vi "sensory_mapping.vi"() -> ()   [LabVIEW 2017]
uses:
  <resource>/objmgr/daqmx.rc
  <vilib>/DAQmx/create/channels.llb/DAQmx Create Channel (DO-Digital Output).vi
  <vilib>/DAQmx/write.llb/DAQmx Write (Digital Bool 1Line 1Point).vi
  const.ctl
  <vilib>/Waveform/WDTOps.llb/WDT Get Waveform Time Array DBL.vi
  <vilib>/DAQmx/read.llb/DAQmx Read (Analog Wfm 1Chan 1Samp).vi
  <vilib>/DAQmx/configure/timing.llb/DAQmx Timing (Sample Clock).vi
  <vilib>/DAQmx/create/channels.llb/DAQmx Create Channel (AI-Voltage-Basic).vi
  <vilib>/Utility/file.llb/Write Delimited Spreadsheet (DBL).vi
  <vilib>/Utility/file.llb/Write Delimited Spreadsheet (string).vi
panel:
  in  "Session":i32=1
  in  "Mouse ID":string
  in  "Base data directory":path
  in  "Stimulated brain region":string
  in  "Vibration Amplitude":dbl
  in  "Vibration frequency (Hz)":dbl
  in  "Simulus duration (seconds)":dbl
  in  "Repeats":i16
  in  "Post_stim (s)":dbl
  in  "Pre_stim (s)":dbl
  in  "Investigator":string
  in  "Stim Type":enum16{"Visual", "Sensory", "Auditory"}(ring)=enum."Sensory"
  in  "Tone Frequency (Hz)":dbl
  out "Stim times":dbl[](array[numeric])
  in  "stop":bool
  out "Current stim iteration":i32
  out "Measured Stim duration (s)":dbl
  in  "Sensory stim output line":tag="Dev3/port1/line3"
  in  "Analog input lines":tag="Dev3/ai0"
  in  "LED output line":tag="Dev3/port1/line1"
  out "Stop time (seconds)":dbl
  out "Stim status":bool
  out "Time from sample clock":dbl
  out "Camera exposure signals":waveform(dbl)(graph)
  out "Sampling rate (Hz)":dbl
  # "Timing parameters"
  # "Stim parameters"
  # "n.b. the params below are changed by the stim box\nthey are not controlled by this VI"
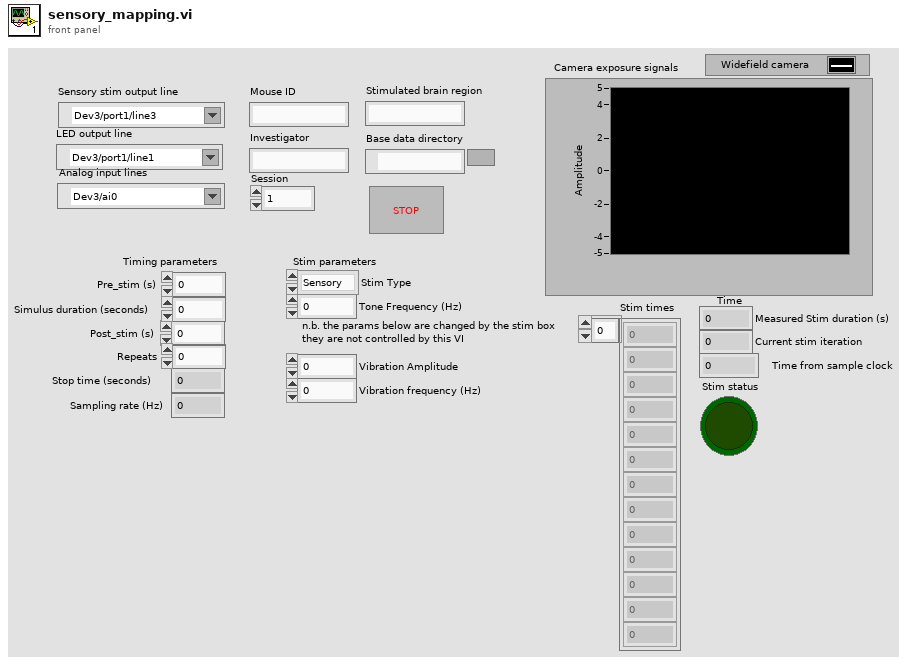
[diagram p1: front panel]
types:
  T1 = cluster{"Mouse ID":string, "Visual Timestamps":dbl[], "Sensory Timestamps":dbl[], "Investigator":string, "Auditory Timestamps":dbl[], "Stim Type":string, "Stop Time":dbl, "Sampling Rate":dbl, "Stimulus Duration (s)":dbl, "Tone Frequency":dbl, "Date_Time":string, "Session":i16, "Synchronisation":dbl[][], "Stimulated brain region":string, "Repeats":i32, "Pre_stim (s)":dbl, "Post_stim (s)":dbl, "Vibration Amplitude":dbl, "Vibration frequency(Hz)":dbl}
  T2 = typedef "const.ctl" = cluster{"Visual":refnum<queue>, "Sensory":refnum<queue>, "Auditory":refnum<queue>}
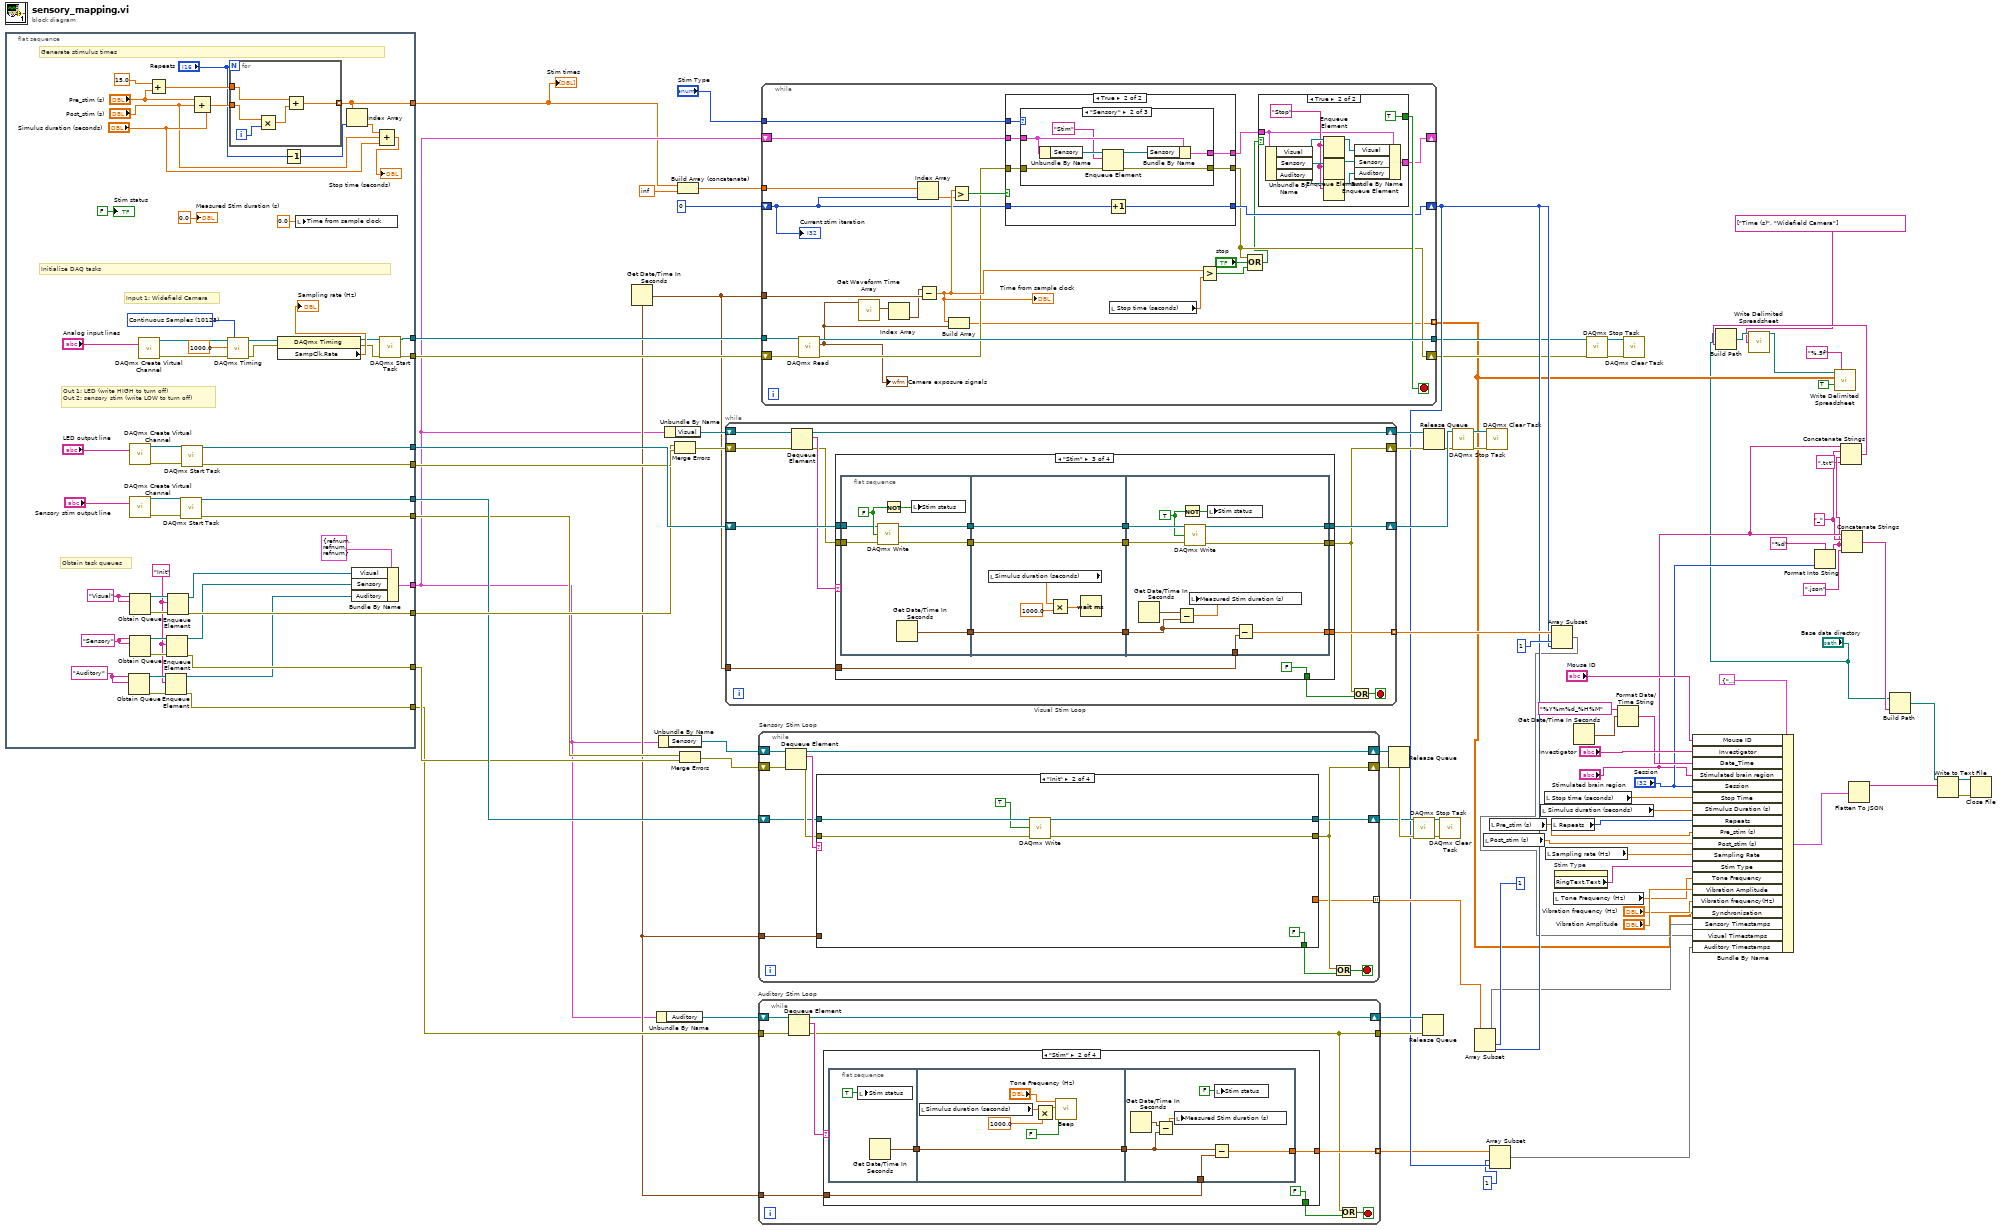
[diagram p0: block diagram]
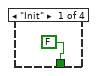
[diagram p2: hidden frame]
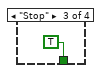
[diagram p3: hidden frame]
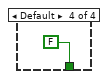
[diagram p4: hidden frame]
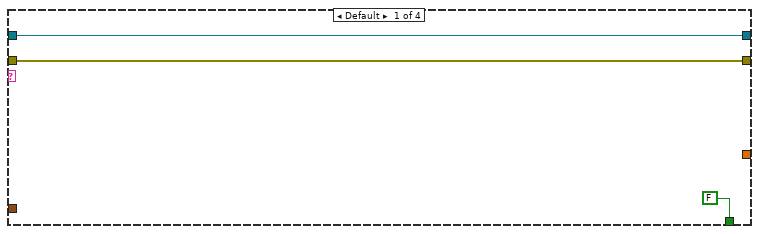
[diagram p5: hidden frame]
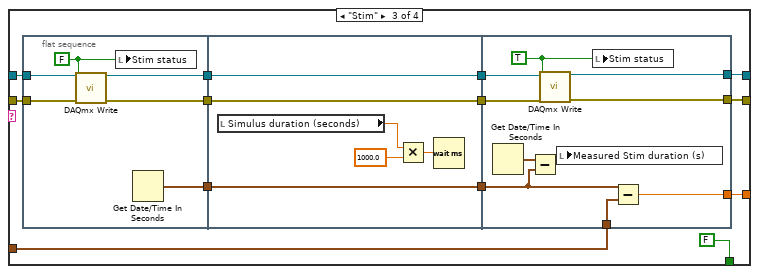
[diagram p6: hidden frame]
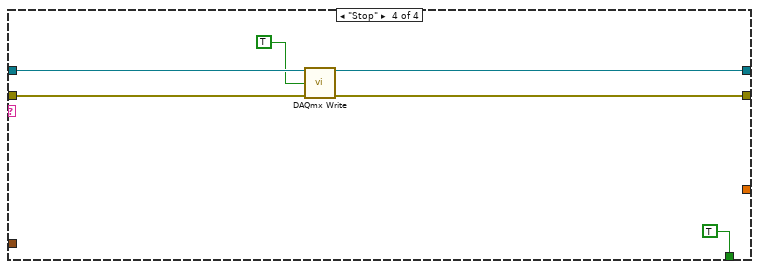
[diagram p7: hidden frame]
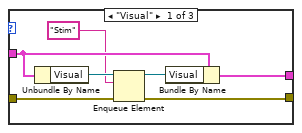
[diagram p9: hidden frame]
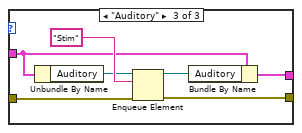
[diagram p10: hidden frame]
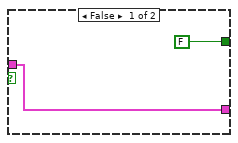
[diagram p11: hidden frame]
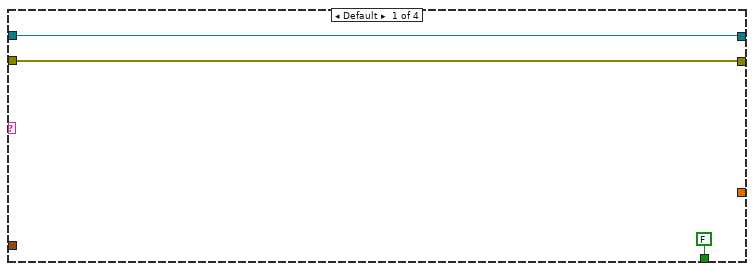
[diagram p12: hidden frame]
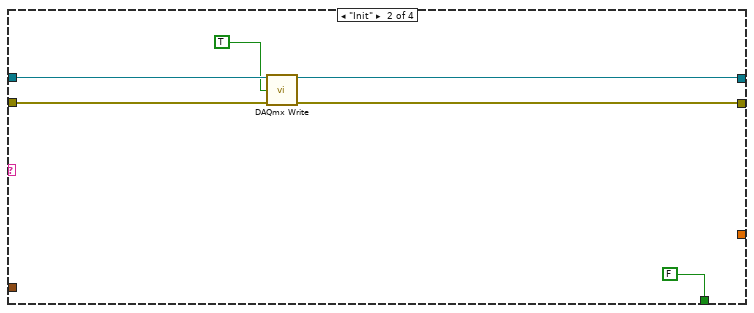
[diagram p13: hidden frame]
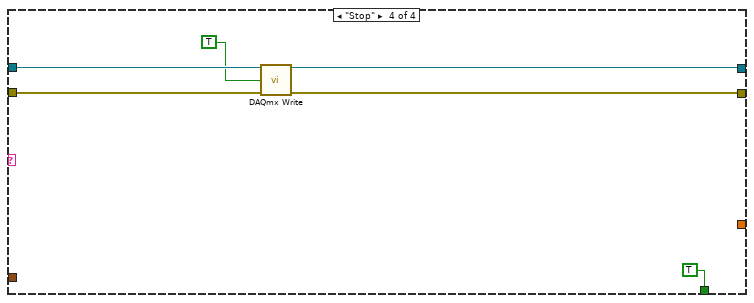
[diagram p14: hidden frame]
diagram:
  w7 = "_" ("string")
  n1 = flat-sequence {
    tunnel: [w127] -> w76
    tunnel: [w126] -> w75
    tunnel: [w122] -> w86
    tunnel: [w121] -> w80
    tunnel: [w117] -> w69
    tunnel: [w109] -> w63
    tunnel: [w108] -> w57
    tunnel: [w103] -> w52
    tunnel: [w102] -> w65
    tunnel: [w101] -> w64
    tunnel: [w93] -> w37
    frame #0 {
      w115 = "Auditory" ("name (unnamed)")
      w116 = "Sensory" ("name (unnamed)")
      w110 = "Init" ("element")
      w118 = "Visual" ("name (unnamed)")
      w138 = 10123 items=["Finite Samples"=10178, "Continuous Samples"=10123, "Hardware Timed Single Point"=12522] ("sample mode")
      # "Generate stimulus times"
      # "Obtain task queues"
      # "Initialize DAQ tasks"
      # "Input 1: Widefield Camera"
      # "Out 1: LED (write HIGH to turn off)\nOut 2: sensory stim (write LOW to turn off)"
      n2 = Obtain Queue(name (unnamed)=w115, element data type=w115) -> (queue out=w112:refnum<queue>, error out=w111:errorcluster)  [unwired: 3 in, 1 out]
      n3 = call-poly <vilib>:"DAQmx Create Virtual Channel.vi"("lines"="LED output line") -> ("task out"=w137:refnum<k21>, "error out"=w136:errorcluster)  [unwired: 13 in]
      n4 = call-poly <vilib>:"DAQmx Create Virtual Channel.vi"("lines"="Sensory stim output line") -> ("task out"=w124:refnum<k21>, "error out"=w123:errorcluster)  [unwired: 13 in]
      n5 = Obtain Queue(name (unnamed)=w118, element data type=w118) -> (queue out=w119:refnum<queue>, error out=w120:errorcluster)  [unwired: 3 in, 1 out]
      n6 = Obtain Queue(name (unnamed)=w116, element data type=w116) -> (queue out=w114:refnum<queue>, error out=w113:errorcluster)  [unwired: 3 in, 1 out]
      n7 = call-poly <vilib>:"DAQmx Create Virtual Channel.vi"("physical channels"="Analog input lines") -> ("task out"=w139:refnum<k21>, "error out"=w140:errorcluster)  [unwired: 13 in]
      n8 = Add(x=15.0, y="Pre_stim (s)") -> (x+y=w94:dbl)
      n9 = Enqueue Element(queue=w112, element=w110, error in (no error)=w111) -> (queue out=w104:refnum<queue>, error out=w108:errorcluster)  [unwired: 1 in, 1 out]
      n10 = Enqueue Element(queue=w114, element=w110, error in (no error)=w113) -> (queue out=w105:refnum<queue>, error out=w109:errorcluster)  [unwired: 1 in, 1 out]
      n11 = Enqueue Element(queue=w119, element=w110, error in (no error)=w120) -> (queue out=w106:refnum<queue>, error out=w117:errorcluster)  [unwired: 1 in, 1 out]
      n12 = call <vilib>:"DAQmx Start Task.vi"("task/channels in"=w124, "error in"=w123) -> ("task out"=w102:refnum<k21>, "error out"=w101:errorcluster)  [unwired: 12 in]
      n13 = call <vilib>:"DAQmx Start Task.vi"("task/channels in"=w137, "error in"=w136) -> ("task out"=w122:refnum<k21>, "error out"=w121:errorcluster)  [unwired: 12 in]
      n14 = Compound Arithmetic op=ADD("Pre_stim (s)", "Post_stim (s)", "Simulus duration (seconds)") -> (w97:dbl)
      n15 = call-poly <vilib>:"DAQmx Timing.vi"("task/channels in"=w139, "sample mode"=w138, "rate"=1000.0, "error in"=w140) -> ("task out"=w132:refnum<k21>, "error out"=w131:errorcluster)  [unwired: 10 in]
      n16 = for {
        N: "Repeats" -> [_]
        tunnel: w97 -> [w144]
        tunnel: w94 -> [w143]
        tunnel: [w141] -> w93 mode=indexing
        i -> [w145]
        n17 = Multiply(x=w144, y=w145) -> (x*y=w142:dbl)
        n18 = Add(x=w143, y=w142) -> (x+y=w141:dbl)
      }
      n19 = property class="DAQmx Timing"(reference=w132, error in=w131) -> (reference out=w129:refnum<k21>, error out=w128:errorcluster, "SampClk.Rate"=→"Sampling rate (Hz)":dbl)
      n20 = Decrement(x="Repeats") -> (x-1=w91:i16)
      n21 = local write "Time from sample clock"(0.0 ("Time from sample clock")) -> ()
      n22 = Index Array(array=w93, index=w91) -> (element=w90:dbl)
      n23 = Bundle By Name(cluster=T2 {"Visual"=refnum, "Sensory"=refnum, "Auditory"=refnum}, "Visual"=w106, "Sensory"=w105, "Auditory"=w104) -> (w103:T2)
      n24 = Compound Arithmetic op=ADD(w90, "Post_stim (s)", "Simulus duration (seconds)") -> (→"Stop time (seconds)":dbl)
      n25 = call <vilib>:"DAQmx Start Task.vi"("task/channels in"=w129, "error in"=w128) -> ("task out"=w127:refnum<k21>, "error out"=w126:errorcluster)  [unwired: 12 in]
      "Stim status" <- FALSE ("LED status")
      "Measured Stim duration (s)" <- 0.0 ("Measured LED duration")
    }
  }
  n26 = Get Date/Time In Seconds() -> (seconds since 1Jan1904=w54:timestamp)
  n27 = Unbundle By Name(w52) -> ("Auditory"=w56:refnum<queue>)
  n28 = Unbundle By Name(w52) -> ("Sensory"=w66:refnum<queue>)
  n29 = Unbundle By Name(w52) -> ("Visual"=w68:refnum<queue>)
  n30 = Merge Errors(w69, w80) -> (w79:errorcluster)
  n31 = Build Array (concatenate)(w37, inf) -> (w74:dbl[])
  n32 = Merge Errors(w64, w63) -> (w62:errorcluster)
  n33 = while "Visual Stim Loop" {
    tunnel: [w157] -> w70 mode=indexing
    shift-right: [w155] -> w81
    shift-left: w86 -> [w156]
    shift-right: [w152] -> w78
    shift-left: w79 -> [w151]
    shift-right: [w146] -> w67
    shift-left: w68 -> [w147]
    tunnel: w54 -> [w148]
    stop <- w154 stop-if-true
    n34 = Dequeue Element(queue=w147, error in (no error)=w151) -> (queue out=w146:refnum<queue>, element=w150:string, error out=w149:errorcluster)  [unwired: 1 in, 1 out]
    n35 = case shown="\"Stim\"" w150 {
      tunnel: [_ _ w173 _] -> w157
      tunnel: w156 -> [w160 w166 w172 w209]
      tunnel: w149 -> [w159 w165 w171 w208]
      tunnel: [w160 w164 w170 w206] -> w155
      tunnel: [w159 w163 w169 w205] -> w152
      tunnel: [FALSE FALSE FALSE TRUE] -> w153
      tunnel: w148 -> [_ _ w167 _]
      frame Default {
      }
      frame "Init" {
        n36 = call-poly <vilib>:"DAQmx Write.vi"("task/channels in"=w166, "data"=TRUE, "error in"=w165) -> ("task out"=w164:refnum<k21>, "error out"=w163:errorcluster)  [unwired: 10 in, 1 out]
      }
      frame "Stim" {
        n37 = flat-sequence {
          tunnel: [w186] -> w179
          tunnel: [w185] -> w178
          tunnel: [w184] -> w177
          tunnel: w172 -> [w181]
          tunnel: w171 -> [w180]
          tunnel: [w190] -> w176
          tunnel: w179 -> [w190]
          tunnel: [w189] -> w175
          tunnel: w178 -> [w189]
          tunnel: [w188] -> w174
          tunnel: w177 -> [w188]
          tunnel: w176 -> [w194]
          tunnel: w175 -> [w202]
          tunnel: w174 -> [w201]
          tunnel: [w193] -> w173
          tunnel: [w197] -> w170
          tunnel: [w196] -> w169
          tunnel: w167 -> [w195]
          frame #0 {
            w183 = FALSE ("data")
            n38 = call-poly <vilib>:"DAQmx Write.vi"("task/channels in"=w181, "data"=w183, "error in"=w180) -> ("task out"=w185:refnum<k21>, "error out"=w184:errorcluster)  [unwired: 10 in, 1 out]
            n39 = Not(x=w183) -> (.not. x?=w182:bool)
            n40 = Get Date/Time In Seconds() -> (seconds since 1Jan1904=w186:timestamp)
            n41 = local write "Stim status"(w182) -> ()
          }
          frame #1 {
            n42 = local read "Simulus duration (seconds)"() -> (w187:dbl)
            n43 = Multiply(x=w187, y=1000.0) -> (x*y=w191:dbl)
            n44 = Wait (ms)(milliseconds to wait=w191) -> ()  [unwired: 1 out]
          }
          frame #2 {
            w200 = TRUE ("data")
            n45 = Get Date/Time In Seconds() -> (seconds since 1Jan1904=w203:timestamp)
            n46 = Subtract(x=w203, y=w194) -> (x-y=w198:dbl)
            n47 = Not(x=w200) -> (.not. x?=w199:bool)
            n48 = call-poly <vilib>:"DAQmx Write.vi"("task/channels in"=w202, "data"=w200, "error in"=w201) -> ("task out"=w197:refnum<k21>, "error out"=w196:errorcluster)  [unwired: 10 in, 1 out]
            n49 = local write "Measured Stim duration (s)"(w198) -> ()
            n50 = local write "Stim status"(w199) -> ()
            n51 = Subtract(x=w194, y=w195) -> (x-y=w193:dbl)
          }
        }
      }
      frame "Stop" {
        n52 = call-poly <vilib>:"DAQmx Write.vi"("task/channels in"=w209, "data"=TRUE, "error in"=w208) -> ("task out"=w206:refnum<k21>, "error out"=w205:errorcluster)  [unwired: 10 in, 1 out]
      }
    }
    n53 = Or(x=w152, y=w153) -> (x .or. y?=w154:bool)
  }
  n54 = while "Auditory Stim Loop" {
    tunnel: w57 -> [w217]
    shift-right: [w216] -> w55
    shift-left: w56 -> [w218]
    tunnel: w54 -> [w214]
    tunnel: [w213] -> w38 mode=indexing
    tunnel: [w210] -> w53
    stop <- w212 stop-if-true
    n55 = Dequeue Element(queue=w218, error in (no error)=w217) -> (queue out=w216:refnum<queue>, element=w215:string, error out=w210:errorcluster)  [unwired: 1 in, 1 out]
    n56 = case shown="\"Stim\"" w215 {
      tunnel: w214 -> [_ w222 _ _]
      tunnel: [_ w221 _ _] -> w213
      tunnel: [FALSE FALSE TRUE FALSE] -> w211
      frame "Init" {
      }
      frame "Stim" {
        n57 = flat-sequence {
          tunnel: [w225] -> w223
          tunnel: [w228] -> w224
          tunnel: w223 -> [w228]
          tunnel: w224 -> [w234]
          tunnel: w222 -> [w236]
          tunnel: [w235] -> w221
          frame #0 {
            n58 = local write "Stim status"(TRUE ("LED status")) -> ()
            n59 = Get Date/Time In Seconds() -> (seconds since 1Jan1904=w225:timestamp)
          }
          frame #1 {
            n60 = local read "Simulus duration (seconds)"() -> (w227:dbl)
            n61 = Multiply(x=w227, y=1000.0) -> (x*y=w231:dbl)
            n62 = call <vilib>:"Beep.vi"("use system alert? (T)"=FALSE, "duration (msec)"=w231, "frequency (Hz)"="Tone Frequency (Hz)") -> ()  [unwired: 9 in]
          }
          frame #2 {
            n63 = Get Date/Time In Seconds() -> (seconds since 1Jan1904=w237:timestamp)
            n64 = Subtract(x=w237, y=w234) -> (x-y=w238:dbl)
            n65 = local write "Measured Stim duration (s)"(w238) -> ()
            n66 = Subtract(x=w234, y=w236) -> (x-y=w235:dbl)
            n67 = local write "Stim status"(FALSE ("LED status")) -> ()
          }
        }
      }
      frame "Stop" {
      }
      frame Default {
      }
    }
    n68 = Or(x=w210, y=w211) -> (x .or. y?=w212:bool)
  }
  n69 = while "Sensory Stim Loop" {
    shift-right: [w251] -> w61
    shift-left: w66 -> [w252]
    shift-right: [w244] -> w60
    shift-left: w62 -> [w249]
    tunnel: w54 -> [w242]
    shift-right: [w246] -> w58
    shift-left: w65 -> [w247]
    tunnel: [w241] -> w49 mode=indexing
    stop <- w245 stop-if-true
    n70 = Dequeue Element(queue=w252, error in (no error)=w249) -> (queue out=w251:refnum<queue>, element=w250:string, error out=w248:errorcluster)  [unwired: 1 in, 1 out]
    n71 = case shown="\"Init\"" w250 {
      tunnel: w248 -> [w254 w261 w272 w301]
      tunnel: w247 -> [w255 w260 w273 w302]
      tunnel: [w255 w259 w267 w300] -> w246
      tunnel: [w254 w258 w266 w299] -> w244
      tunnel: [FALSE FALSE FALSE TRUE] -> w243
      tunnel: w242 -> [_ _ w274 _]
      tunnel: [_ _ w262 _] -> w241
      frame Default {
      }
      frame "Init" {
        n72 = call-poly <vilib>:"DAQmx Write.vi"("task/channels in"=w260, "data"=TRUE, "error in"=w261) -> ("task out"=w259:refnum<k21>, "error out"=w258:errorcluster)  [unwired: 10 in, 1 out]
      }
      frame "Stim" {
        n73 = flat-sequence {
          tunnel: w273 -> [w280]
          tunnel: w272 -> [w279]
          tunnel: [w277] -> w270
          tunnel: [w276] -> w268
          tunnel: [w275] -> w263
          tunnel: [w286] -> w271
          tunnel: w270 -> [w286]
          tunnel: [w285] -> w269
          tunnel: w268 -> [w285]
          tunnel: [w282] -> w264
          tunnel: w263 -> [w282]
          tunnel: w274 -> [w288]
          tunnel: w271 -> [w296]
          tunnel: w269 -> [w295]
          tunnel: [w293] -> w267
          tunnel: [w292] -> w266
          tunnel: w264 -> [w289]
          tunnel: [w287] -> w262
          frame #0 {
            w278 = FALSE ("data")
            n74 = call-poly <vilib>:"DAQmx Write.vi"("task/channels in"=w280, "data"=w278, "error in"=w279) -> ("task out"=w277:refnum<k21>, "error out"=w276:errorcluster)  [unwired: 10 in, 1 out]
            n75 = local write "Stim status"(w278) -> ()
            n76 = Get Date/Time In Seconds() -> (seconds since 1Jan1904=w275:timestamp)
          }
          frame #1 {
            n77 = local read "Simulus duration (seconds)"() -> (w281:dbl)
            n78 = Multiply(x=w281, y=1000.0) -> (x*y=w284:dbl)
            n79 = Wait (ms)(milliseconds to wait=w284) -> ()  [unwired: 1 out]
          }
          frame #2 {
            w294 = TRUE ("data")
            n80 = Get Date/Time In Seconds() -> (seconds since 1Jan1904=w290:timestamp)
            n81 = Subtract(x=w290, y=w289) -> (x-y=w291:dbl)
            n82 = call-poly <vilib>:"DAQmx Write.vi"("task/channels in"=w296, "data"=w294, "error in"=w295) -> ("task out"=w293:refnum<k21>, "error out"=w292:errorcluster)  [unwired: 10 in, 1 out]
            n83 = local write "Measured Stim duration (s)"(w291) -> ()
            n84 = local write "Stim status"(w294) -> ()
            n85 = Subtract(x=w289, y=w288) -> (x-y=w287:dbl)
          }
        }
      }
      frame "Stop" {
        n86 = call-poly <vilib>:"DAQmx Write.vi"("task/channels in"=w302, "data"=TRUE, "error in"=w301) -> ("task out"=w300:refnum<k21>, "error out"=w299:errorcluster)  [unwired: 10 in, 1 out]
      }
    }
    n87 = Or(x=w244, y=w243) -> (x .or. y?=w245:bool)
  }
  n88 = while {
    tunnel: w54 -> [w327]
    tunnel: w76 -> [w324]
    tunnel: [w322] -> w20
    shift-right: [w310] -> _
    shift-left: w52 -> [w313]
    tunnel: w74 -> [w318]
    shift-right: [w315] -> w40
    shift-left: 0 ("Current LED iteration") -> [w316]
    tunnel: "Stim Type" -> [w314]
    shift-right: [w309] -> w19
    shift-left: w75 -> [w323]
    tunnel: [w305] -> w11 mode=indexing
    stop <- w321 stop-if-true
    n89 = call-poly <vilib>:"DAQmx Read.vi"("task/channels in"=w324, "error in"=w323) -> ("task out"=w322:refnum<k21>, "data"=w304:waveform(dbl), "error out"=w312:errorcluster)  [unwired: 11 in]
    "Camera exposure signals" <- w304
    n90 = call-poly <vilib>:"Get Waveform Time Array.vi"("waveform in"=w304) -> ("X array"=w326:timestamp[])  [unwired: 9 in, 1 out]
    n91 = Index Array(array=w326) -> (element=w325:timestamp)  [unwired: 1 in]
    n92 = Index Array(array=w318, index=w316) -> (element=w319:dbl)
    n93 = Subtract(x=w325, y=w327) -> (x-y=w320:dbl)
    "Time from sample clock" <- w320
    n94 = Build Array(w320, w304) -> (w305:dbl[])
    n95 = Greater?(x=w320, y=w319) -> (0:w317:bool)
    n96 = case shown="True" w317 {
      tunnel: w313 -> [w330 w334]
      tunnel: [w330 w333] -> w311
      tunnel: w316 -> [w329 w337]
      tunnel: [w329 w336] -> w315
      tunnel: w314 -> [_ w335]
      tunnel: w312 -> [w328 w332]
      tunnel: [w328 w331] -> w309
      frame False {
      }
      frame True {
        n97 = case shown="\"Sensory\"" w335 {
          tunnel: w334 -> [w342 w348 w355]
          tunnel: [w340 w349 w358] -> w333
          tunnel: w332 -> [w339 w346 w353]
          tunnel: [w338 w345 w352] -> w331
          frame "Visual" {
            n98 = Unbundle By Name(w342) -> ("Visual"=w344:refnum<queue>)
            n99 = Enqueue Element(queue=w344, element="Stim", error in (no error)=w339) -> (queue out=w343:refnum<queue>, error out=w338:errorcluster)  [unwired: 1 in, 1 out]
            n100 = Bundle By Name(cluster=w342, "Visual"=w343) -> (w340:T2)
          }
          frame "Sensory" {
            n101 = Unbundle By Name(w348) -> ("Sensory"=w351:refnum<queue>)
            n102 = Enqueue Element(queue=w351, element="Stim", error in (no error)=w346) -> (queue out=w350:refnum<queue>, error out=w345:errorcluster)  [unwired: 1 in, 1 out]
            n103 = Bundle By Name(cluster=w348, "Sensory"=w350) -> (w349:T2)
          }
          frame "Auditory" {
            n104 = Unbundle By Name(w355) -> ("Auditory"=w356:refnum<queue>)
            n105 = Enqueue Element(queue=w356, element="Stim", error in (no error)=w353) -> (queue out=w354:refnum<queue>, error out=w352:errorcluster)  [unwired: 1 in, 1 out]
            n106 = Bundle By Name(cluster=w355, "Auditory"=w354) -> (w358:T2)
          }
        }
        n107 = Increment(x=w337) -> (x+1=w336:i32)
      }
    }
    n108 = local read "Stop time (seconds)"() -> (w303:dbl)
    n109 = Greater?(x=w320, y=w303) -> (0:w307:bool)
    n110 = Compound Arithmetic op=OR(w309, "stop", w307) -> (w306:bool)
    n111 = case shown="True" w306 {
      tunnel: [FALSE TRUE] -> w321
      tunnel: w311 -> [w359 w362]
      tunnel: [w359 w361] -> w310
      frame False {
      }
      frame True {
        w366 = "Stop" ("element")
        n112 = Unbundle By Name(w362) -> ("Visual"=w369:refnum<queue>, "Sensory"=w368:refnum<queue>, "Auditory"=w367:refnum<queue>)
        n113 = Enqueue Element(queue=w369, element=w366) -> (queue out=w365:refnum<queue>)  [unwired: 2 in, 2 out]
        n114 = Enqueue Element(queue=w368, element=w366) -> (queue out=w364:refnum<queue>)  [unwired: 2 in, 2 out]
        n115 = Enqueue Element(queue=w367, element=w366) -> (queue out=w363:refnum<queue>)  [unwired: 2 in, 2 out]
        n116 = Bundle By Name(cluster=w362, "Visual"=w365, "Sensory"=w364, "Auditory"=w363) -> (w361:T2)
      }
    }
    "Current stim iteration" <- w316
  }
  n117 = Release Queue(queue=w61, error in (no error)=w60) -> (error out=w59:errorcluster)  [unwired: 1 in, 2 out]
  n118 = call <vilib>:"DAQmx Stop Task.vi"("task/channels in"=w58, "error in"=w59) -> ("task out"=w85:refnum<k21>, "error out"=w84:errorcluster)  [unwired: 12 in]
  n119 = Release Queue(queue=w55, error in (no error)=w53) -> ()  [unwired: 1 in, 3 out]
  n120 = Release Queue(queue=w67, error in (no error)=w78) -> (error out=w77:errorcluster)  [unwired: 1 in, 2 out]
  n121 = call <vilib>:"DAQmx Clear Task.vi"("task in"=w85, "error in"=w84) -> ()  [unwired: 13 in, 1 out]
  n122 = call <vilib>:"DAQmx Stop Task.vi"("task/channels in"=w81, "error in"=w77) -> ("task out"=w83:refnum<k21>, "error out"=w82:errorcluster)  [unwired: 12 in]
  n123 = Array Subset(array=w49, index=1, length=w40) -> (w14:dbl[])
  n124 = local read "Post_stim (s)"() -> (w23:dbl)
  n125 = call <vilib>:"DAQmx Clear Task.vi"("task in"=w83, "error in"=w82) -> ()  [unwired: 13 in, 1 out]
  n126 = local read "Pre_stim (s)"() -> (w24:dbl)
  n127 = Array Subset(array=w38, index=1, length=w40) -> (w36:dbl[])
  n128 = local read "Simulus duration (seconds)"() -> (w29:dbl)
  n129 = local read "Stop time (seconds)"() -> (w30:dbl)
  n130 = local read "Sampling rate (Hz)"() -> (w31:dbl)
  n131 = Array Subset(array=w70, index=1, length=w40) -> (w13:dbl[])
  n132 = local read "Repeats"() -> (w28:i16)
  n133 = local read "Tone Frequency (Hz)"() -> (w33:dbl)
  n134 = property on="Stim Type" class="Enum (strict)"() -> ("RingText.Text"=w32:string)  [unwired: 2 in, 2 out]
  n135 = Get Date/Time In Seconds() -> (seconds since 1Jan1904=w45:timestamp)
  n136 = call <vilib>:"DAQmx Stop Task.vi"("task/channels in"=w20, "error in"=w19) -> ("task out"=w21:refnum<k21>, "error out"=w22:errorcluster)  [unwired: 12 in]
  n137 = Format Date/Time String(time format string (%c)="%Y%m%d_%H%M", seconds (now)=w45) -> (date/time string=w26:string)  [unwired: 1 in]
  n138 = call <vilib>:"DAQmx Clear Task.vi"("task in"=w21, "error in"=w22) -> ()  [unwired: 13 in, 1 out]
  n139 = Bundle By Name(cluster=T1 {"Mouse ID"="TEST", "Visual Timestamps"=[], "Sensory Timestamps"=[], "Investigator"="MP", "Auditory Timestamps"=[], "Stim Type"="TEST", "Stop Time"=0.0, "Sampling Rate"=0.0, "Stimulus Duration (s)"=0.0, "Tone Frequency"=0.0, "Date_Time"="Today", "Session"=0, "Synchronisation"=[], "Stimulated brain region"="TEST", "Repeats"=0, "Pre_stim (s)"=0.0, "Post_stim (s)"=0.0, "Vibration Amplitude"=0.0, "Vibration frequency(Hz)"=0.0}, "Mouse ID"="Mouse ID", "Investigator"="Investigator", "Date_Time"=w26, "Stimulated brain region"="Stimulated brain region", "Session"="Session", "Stop Time"=w30, "Stimulus Duration (s)"=w29, "Repeats"=w28, "Pre_stim (s)"=w24, "Post_stim (s)"=w23, "Sampling Rate"=w31, "Stim Type"=w32, "Tone Frequency"=w33, "Vibration Amplitude"="Vibration Amplitude", "Vibration frequency(Hz)"="Vibration frequency (Hz)", "Synchronisation"=w11, "Sensory Timestamps"=w14, "Visual Timestamps"=w13, "Auditory Timestamps"=w36) -> (w47:T1)
  n140 = Format Into String(format string="%d", "Session") -> (resulting string=w6:string)  [unwired: 2 in, 1 out]
  n141 = Concatenate Strings("Stimulated brain region", w7, w6, ".txt" ("string")) -> (w4:string)
  n142 = Build Path(base path="Base data directory", name or relative path=w4) -> (appended path=w2:path)
  n143 = call-poly <vilib>:"Write Delimited Spreadsheet.vi"("file path (dialog if empty)"=w2, "1D data"=string[] ["Time (s)", "Widefield Camera"]) -> ("new file path (Not A Path if cancelled)"=w9:path)  [unwired: 12 in, 1 out]
  n144 = call-poly <vilib>:"Write Delimited Spreadsheet.vi"("file path (dialog if empty)"=w9, "format (%.3f)"="%.5f", "2D data"=w11, "append to file? (new file:F)"=TRUE) -> ()  [unwired: 10 in, 2 out]
  n145 = Concatenate Strings("Stimulated brain region", w7, w6, ".json" ("string")) -> (w15:string)
  n146 = Flatten To JSON(anything=w47) -> (JSON string=w43:string)  [unwired: 2 in, 1 out]
  n147 = Build Path(base path="Base data directory", name or relative path=w15) -> (appended path=w44:path)
  n148 = Write to Text File(file (use dialog)=w44, text=w43) -> (refnum out=w41:refnum<file>, error out=w42:errorcluster)  [unwired: 2 in, 1 out]
  n149 = Close File(refnum=w41, error in=w42) -> ()  [unwired: 2 out]
  "Stim times" <- w37
